vi "Actor Core.vi"(8 "error in":errorcluster, 11 "Work Dispatcher in":refnum<class "Work Dispatcher.lvclass">) -> (0 "error out":errorcluster, 3 "Actor out":refnum<class "Actor.lvclass">)   [LabVIEW 2023, in "Work Dispatcher.lvlib" / "Work Dispatcher.lvclass"]
doc: "(<B>Filename</B>: Actor Framework.lvlib:Actor.lvclass:Actor Core.vi)\n\nReceives messages to the actor, reacts to them, and initiates any error handling that may shut the actor down.\n\nDescendant classes may override this VI to append parallel tasks for the actor to complete while it handles messages. Overrides use the Call Parent Method node."
uses:
  Work Dispatcher.lvclass
  <vilib>/ActorFramework/Actor/Actor.lvclass
  <vilib>/ActorFramework/Message Enqueuer/Message Enqueuer.lvclass
  Work Dispatcher.lvclass/Work Dispatcher.ctl
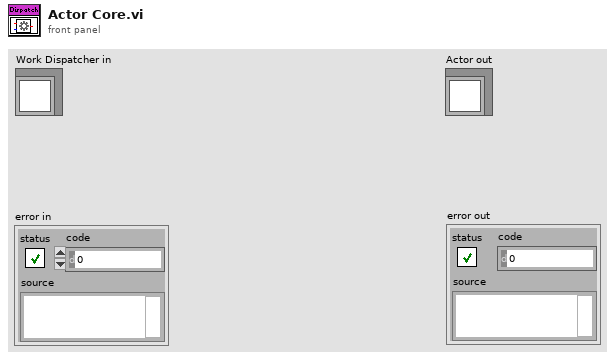
[diagram p1: front panel]
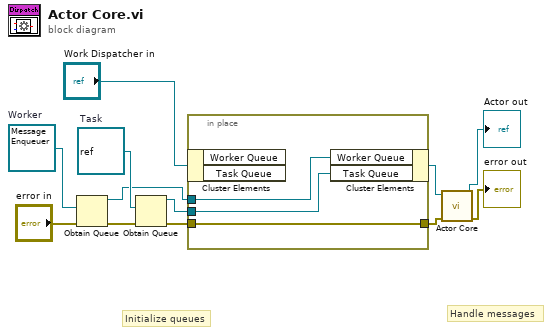
[diagram p0: block diagram]
diagram:
  w8 = refnum<class "Message Enqueuer.lvclass"> refnum  # Worker
  w10 = refnum<class> refnum  # Task
  # "Handle messages"
  # "Initialize queues"
  n1 = Obtain Queue(element data type=w8, error in (no error)="error in") -> (queue out=w7:refnum<queue>, error out=w12:errorcluster)  [unwired: 3 in, 1 out]
  n2 = Obtain Queue(element data type=w10, error in (no error)=w12) -> (queue out=w9:refnum<queue>, error out=w6:errorcluster)  [unwired: 3 in, 1 out]
  n3 = in-place {
    in-place-border: w9 -> [w15]
    in-place-border: w7 -> [w14]
    in-place-border: w6 -> [w13]
    in-place-border: [w13] -> w4
    n4 = in-place-cluster #1("Work Dispatcher in") -> ()  [unwired: 2 out]
    n5 = in-place-cluster #1("Worker Queue"=w14, "Task Queue"=w15) -> (w1:refnum<class "Work Dispatcher.lvclass">)
  }
  n6 = call-parent "Actor Core.vi"("error in"=w4, "Actor in"=w1) -> ("error out"=→"error out":errorcluster, "Actor out"=→"Actor out":refnum<class "Actor.lvclass">)  [unwired: 8 in]
